vi "set_ref_clus_LJU3.vi"(6 "cluster_ref":T2, 9 "Temperature":T1=enum."UNKNOWN", 11 "status":bool) -> ()   [LabVIEW 2019]
uses:
  cluster_ref_LabJackU3.ctl
  temperature_status_LabJackU3.ctl
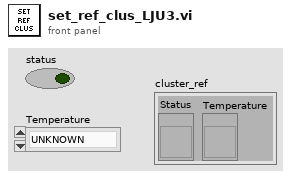
[diagram p1: front panel]
types:
  T1 = typedef "temperature_status_LabJackU3.ctl" = enum16{"OK", "UNKNOWN", "WARNING", "ERROR"}
  T2 = typedef "cluster_ref_LabJackU3.ctl" = cluster{"Status":refnum<vi>, "Temperature":refnum<vi>}
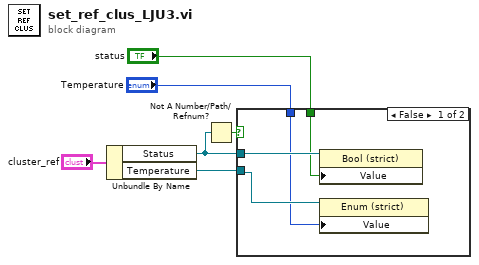
[diagram p0: block diagram]
diagram:
  n1 = Unbundle By Name("cluster_ref") -> ("Status"=w5:refnum<vi>, "Temperature"=w4:refnum<vi>)
  n2 = Not A Number/Path/Refnum?(number/path/refnum=w5) -> (NaN/Path/Refnum?=w6:bool)
  n3 = case shown="False" w6 {
    tunnel: w5 -> [w10 _]
    tunnel: w4 -> [w8 _]
    tunnel: "status" -> [w9 _]
    tunnel: "Temperature" -> [w7 _]
    frame False {
      n4 = property class="Bool (strict)"(reference=w10, "Value"=w9) -> ()  [unwired: 1 in, 2 out]
      n5 = property on="Property Node" class="Enum (strict)"(reference=w8, "Value"=w7) -> ()  [unwired: 1 in, 2 out]
    }
    frame True {
    }
  }
